vi "Check_Execution_Row.vi"(0 "Execution Row":T1 {"Row Duration (mins)" format="%#.1f"; "Row No" min=0; "Trace Gas Concentration (%)" min=0.0 format="%#.2f"; "Emission Rate (l/min)" format="%#.2f"; "Tunnel Speed" format="%#.2f"; "Start X" format="%#.2f"; "Start Y" format="%#.2f"; "Start Z" format="%#.2f"; "End X" format="%#.2f"; "End Y" format="%#.2f"; "End Z" format="%#.2f"; "Averaging time (min)" min=0.0 format="%#.2f"}, 3 "Synchronization Start No":i32=1 min=1 max=100, 4 "Row Index":i32, 5 "Max Tunnel Speed":dbl format="%.2f") -> (6 "Editted Row":bool, 7 "Execution Row Out":T1 {"Row Duration (mins)" format="%#.1f"; "Row No" min=0; "Trace Gas Concentration (%)" min=0.0 format="%#.2f"; "Emission Rate (l/min)" format="%#.2f"; "Tunnel Speed" format="%#.2f"; "Start X" format="%#.2f"; "Start Y" format="%#.2f"; "Start Z" format="%#.2f"; "End X" format="%#.2f"; "End Y" format="%#.2f"; "End Z" format="%#.2f"; "Averaging time (min)" min=0.0 format="%#.2f"}, 9 "Continue?":bool, 10 "Error Comments":string)   [LabVIEW 2010]
uses:
  Traverse_cluster.ctl
  Spacing.ctl
  Controls/Multi_run_mode.ctl
  Controls/User_Specific_mode.ctl
  Controls/Tunnel_Coordinates.ctl
  ADAM Client/Sub VIs/ADAM Controls/Channel_names.ctl
  Globals/Extra_Commands_Global.vi
  Globals/Constants_global.vi
  Globals/Trav_pos_global.vi
panel:
  out "Fixed Axis":bool[](array[boolean])
  out "Filenames":string[](array[string])
  out "Current Sync Number":i32
  out "Checks":string[](array[string])
  in  "Edit in Excel":bool
  in  "OK":bool
  # "X           Y            Z"
  # "Start"
  # "End"
  # "X           Y            Z"
  # "Start"
  # "End"
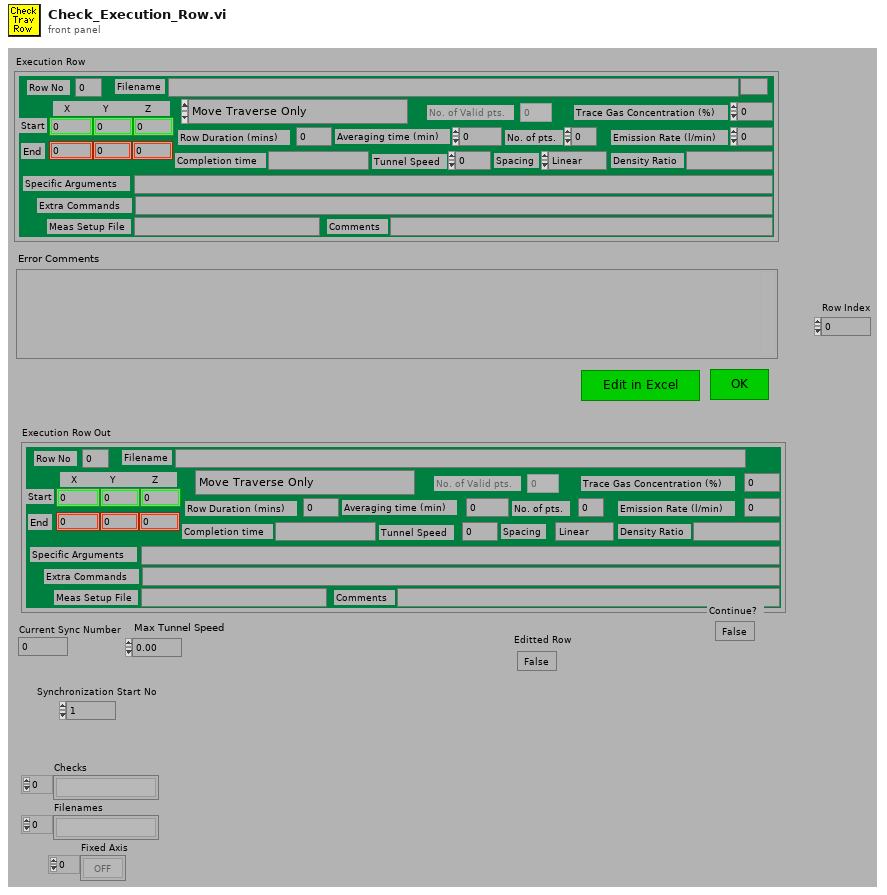
[diagram p1: front panel]
types:
  T1 = typedef "Traverse_cluster.ctl" = cluster{"Start X":dbl, "Start Y":dbl, "Start Z":dbl, "End X":dbl, "End Y":dbl, "End Z":dbl, "No. of pts.":i32, "Spacing":T2, "Filename":path, "Tunnel Speed":dbl, "Averaging time (min)":dbl, "Extra Commands":string, "Specific Arguments":string, "Emission Rate (l/min)":dbl, "Trace Gas Concentration (%)":dbl, "Density Ratio":string, "Comments":string, "Row No":i32, "Row Type Selector":T3, "Completion time":string, "Row Duration (mins)":dbl, "No. of Valid pts.":i32, "Meas Setup File":string}
  T2 = typedef "Spacing.ctl" = enum16{"Linear", "Log", "Gauss", "Specified", "N/A"}
  T3 = typedef "Multi_run_mode.ctl" = enum16{"Move Traverse Only", "Set Tunnel Speed Only", "Set Source Only", "Set Measurement Conditions", "Single Measurement", "Vertical Profile", "Lateral Profile", "Longitudinal Profile", "Explore Volume", "Multi-Axis Profile", "Auto Calibrate", "Meas Fast FID Bkgnd", "Check Beam Power", "Scanning Valve Measurement", "Run VI Named:", "Set ADAM Ch", "Wait (minutes)", "Send Message", "Synchronize With:", "Fall Back to this Row", "Turn Off Row Repeating", "Blank Row"}
  T4 = enum16{"All Channel Names", "Valid Channel Names"}
  T5 = typedef "User_Specific_mode.ctl" = enum16{"Check VI only", "Run VI"}
  T6 = typedef "Tunnel_Coordinates.ctl" = enum16{"Work in Tunnel Coordinates", "Work in Model Coordinates"}
  T7 = enum16{"Zero or one", "One", "Zero or more", "One or more"}
  T8 = typedef "Channel_names.ctl" = enum16{"Active Only", "Active + Off", "All Channels"}
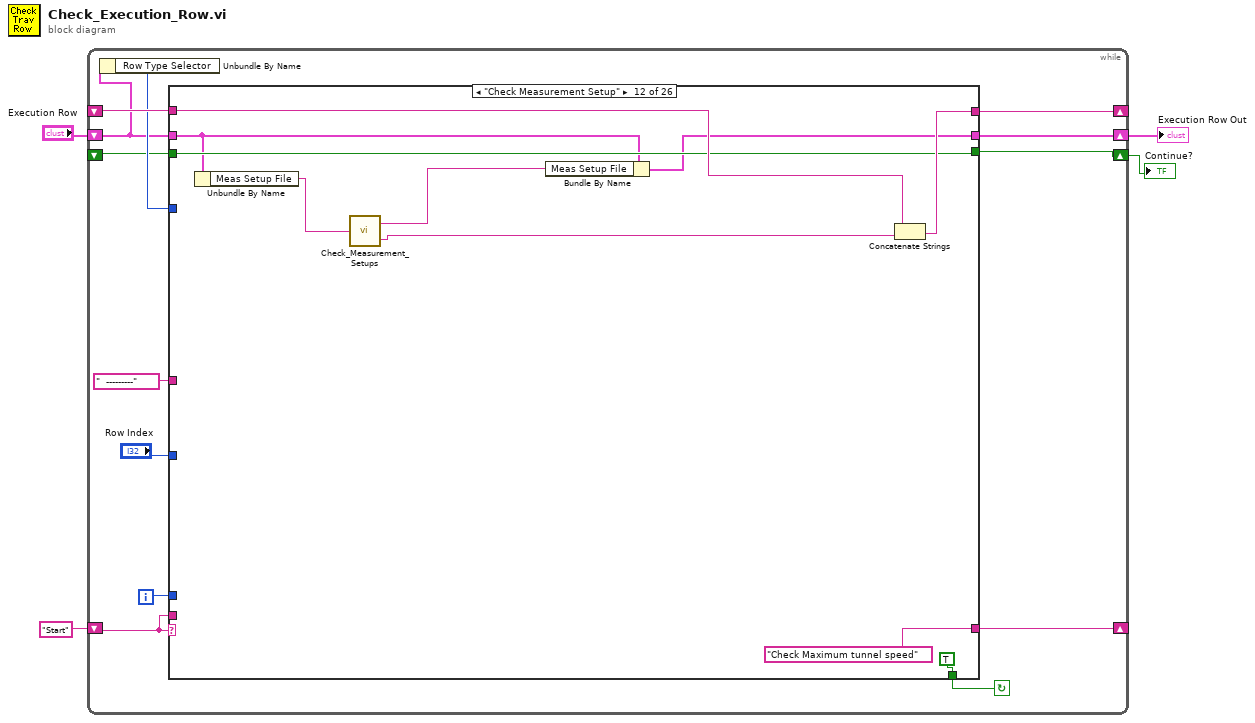
[diagram p0: block diagram]
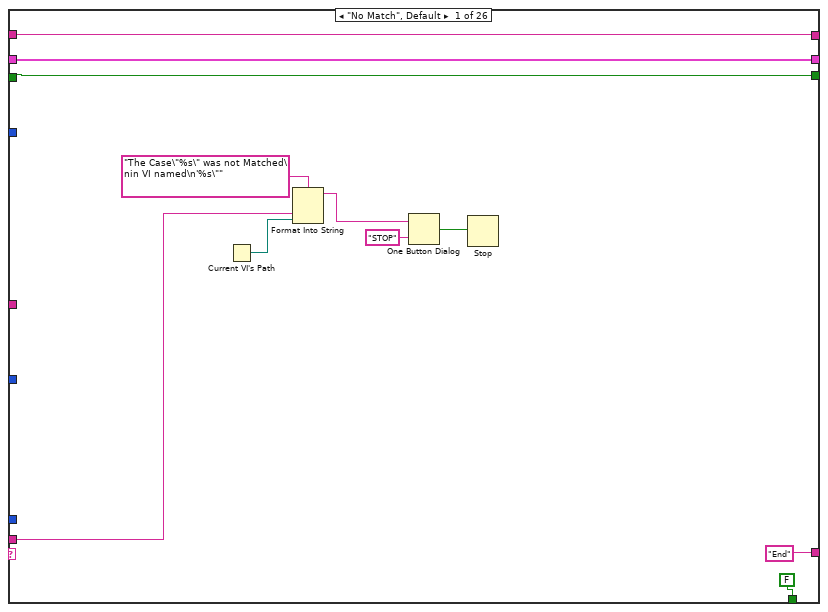
[diagram p2: hidden frame]
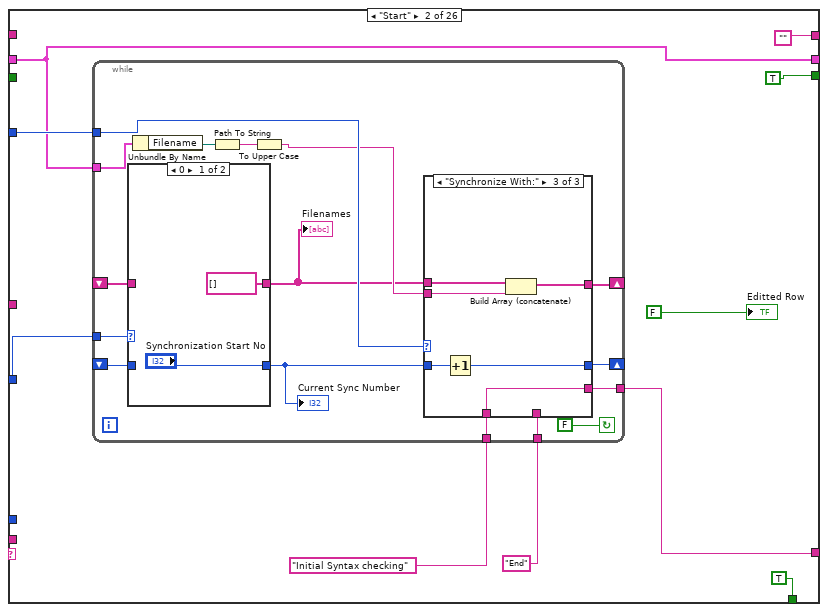
[diagram p3: hidden frame]
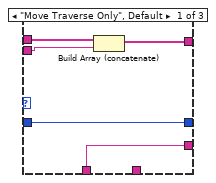
[diagram p5: hidden frame]
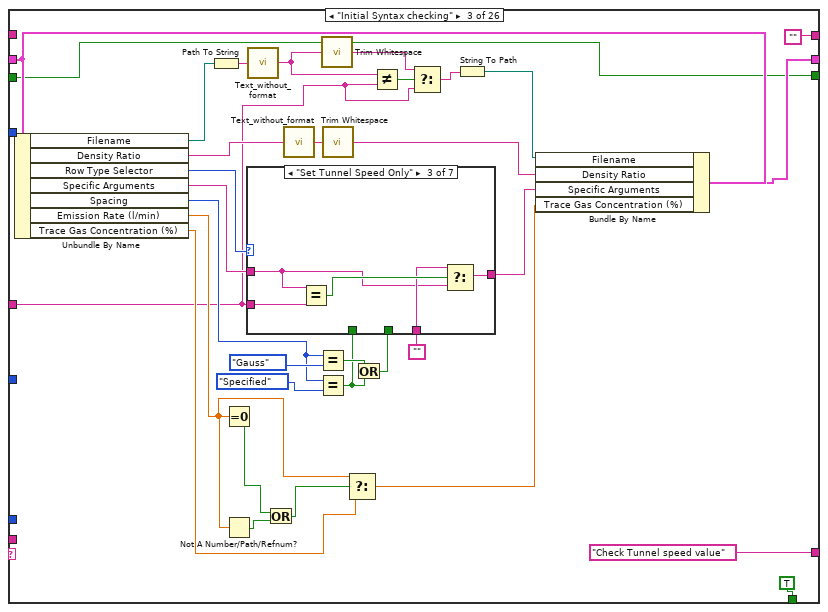
[diagram p7: hidden frame]
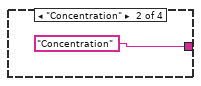
[diagram p10: hidden frame]
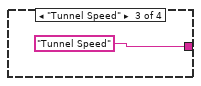
[diagram p11: hidden frame]
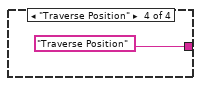
[diagram p12: hidden frame]
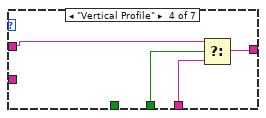
[diagram p13: hidden frame]
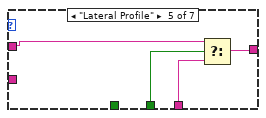
[diagram p14: hidden frame]
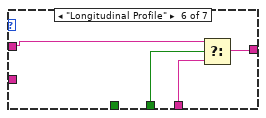
[diagram p15: hidden frame]
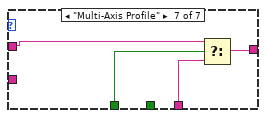
[diagram p16: hidden frame]
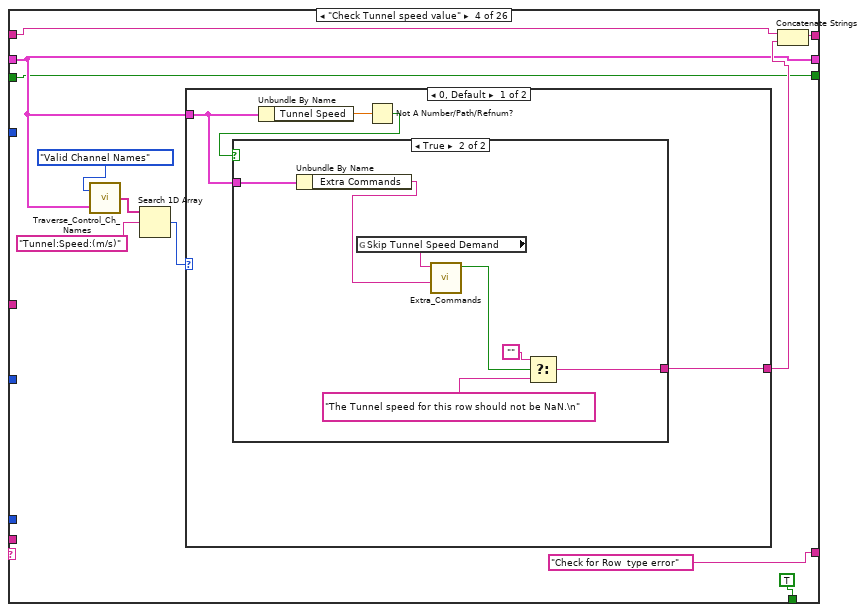
[diagram p17: hidden frame]
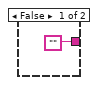
[diagram p18: hidden frame]
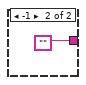
[diagram p19: hidden frame]
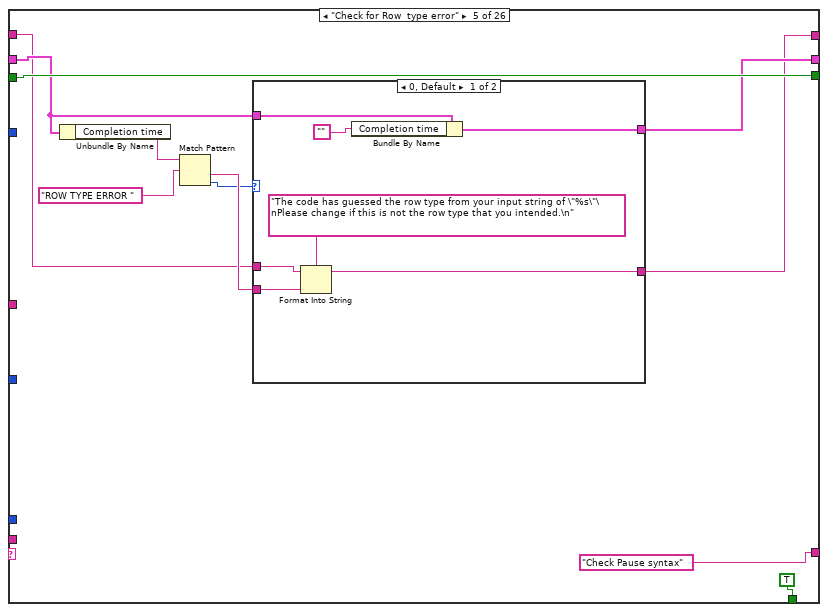
[diagram p20: hidden frame]
diagram:
  n1 = while {
    shift-left: _ -> [w16]
    shift-right: [w17] -> _
    shift-left: "Start" -> [w9]
    shift-right: [w14] -> _
    shift-right: [w8] -> w2
    shift-left: "Execution Row" -> [w5]
    shift-right: [w7] -> w1
    shift-left: _ -> [w6]
    i -> [w10]
    stop <- w15 continue-if-true
    n2 = Unbundle By Name(w5) -> ("Row Type Selector"=w12:T3)
    n3 = case shown="\"Check Measurement Setup\"" w9 {
      tunnel: w5 -> [w22 w32 w100 w137 w161 w191 w204 w252 w283 w313 w369 w401 w409 w448 w779 w879 w916 w938 w1022 w1054 w1064 w1133 _ w1172 w1179 w1189]
      tunnel: "  ---------" ("f") -> [_ _ w74 _ _ w195 _ _ _ _ _ _ _ _ _ _ _ _ _ _ _ _ _ _ _ _]
      tunnel: "Row Index" -> [_ w36 _ _ _ _ w201 _ _ _ _ _ _ w442 _ _ _ _ _ _ _ _ _ w1173 _ w1188]
      tunnel: [w21 "" "" w138 w158 w183 w218 w254 w288 w318 w371 w405 w414 w452 w784 w889 w922 w963 w1020 w1058 w1065 w1139 w1150 w1174 w1184 w1191] -> w17
      tunnel: w12 -> [_ w35 _ _ _ _ w209 _ _ _ _ _ w412 w451 w780 w877 _ _ _ _ w1069 _ _ _ _ _]
      tunnel: w16 -> [w21 _ _ w139 w159 w185 w219 w255 w289 w319 w371 w404 w415 w453 w784 w890 w923 w964 w1020 w1059 w1070 w1139 w1150 w1174 w1184 w1191]
      tunnel: [FALSE TRUE TRUE TRUE TRUE TRUE TRUE TRUE TRUE TRUE TRUE TRUE TRUE TRUE TRUE TRUE TRUE TRUE TRUE TRUE w1061 TRUE TRUE TRUE TRUE FALSE] -> w15
      tunnel: ["End" w33 "Check Tunnel speed value" ("f") "Check for Row  type error" ("f") "Check Pause syntax" ("f") w188 w206 "Check Traverse Setup Name" ("f") "Check IF command" ("f") "Check Measurement Setup?" ("f") w373 "Check Maximum tunnel speed" ("f") "Row type specific check" ("f") w449 "Check for position NaNs" ("f") w880 "Check source details" ("t") "Check source details" ("f") w1017 "check entered filename etc" ("f") w1067 "What to do next?" ("f") w1148 "Initial Syntax checking" "End" "End"] -> w14
      tunnel: w10 -> [_ _ _ _ _ _ _ _ _ _ _ _ _ _ _ _ _ _ _ _ _ _ _ _ _ _]
      tunnel: w9 -> [w23 _ _ _ _ _ _ _ _ _ _ _ _ _ _ _ _ _ _ _ _ _ _ _ _ _]
      tunnel: [w22 w32 w77 w137 w162 w178 w203 w252 w283 w313 w369 w400 w409 w443 w778 w879 w916 w937 w1021 w1054 w1063 w1133 w1141 w1175 w1179 w1187] -> w8
      tunnel: [w18 TRUE w75 w136 w168 w179 w205 w248 w280 w310 w375 w402 w407 w445 w776 w878 w915 w935 w1025 w1052 w1061 w1132 w1140 w1169 w1178 w1185] -> w7
      tunnel: w6 -> [w18 _ w75 w136 w168 w179 w205 w248 w280 w310 w375 w402 w407 w445 w776 w878 w915 w935 w1025 w1052 _ w1132 _ w1169 w1178 w1185]
      frame "No Match", Default {
        n4 = Current VI's Path() -> (path=w24:path)
        n5 = Format Into String(format string="The Case\"%s\" was not Matched\nin VI named\n'%s\"" ("Format String"), w23, w24) -> (resulting string=w27:string)  [unwired: 2 in, 1 out]
        n6 = One Button Dialog(message=w27, button name ("OK")="STOP") -> (true=w25:bool)
        n7 = Stop(stop? (T)=w25) -> ()
      }
      frame "Start" {
        n8 = while {
          tunnel: "End" -> [w40]
          tunnel: "Initial Syntax checking" -> [w41]
          tunnel: [w42] -> w33
          tunnel: w32 -> [w49]
          shift-left: _ -> [w48]
          shift-right: [w47] -> _
          tunnel: w35 -> [w53]
          shift-left: _ -> [w52]
          shift-right: [w51] -> _
          tunnel: w36 -> [w54]
          stop <- FALSE continue-if-true
          n9 = case shown="0" w54 {
            tunnel: ["Synchronization Start No" w58] -> w50
            tunnel: w52 -> [_ w58]
            tunnel: w48 -> [_ w57]
            tunnel: [string[] [] w57] -> w43
            frame 0 {
            }
            frame 1, Default {
            }
          }
          "Current Sync Number" <- w50
          "Filenames" <- w43
          n10 = Unbundle By Name(w49) -> ("Filename"=w46:path)
          n11 = Path To String(path=w46) -> (string=w45:string)
          n12 = To Upper Case(1:w45) -> (0:w44:string)
          n13 = case shown="\"Synchronize With:\"" w53 {
            tunnel: w50 -> [w63 w66 w72]
            tunnel: [w63 w66 w71] -> w51
            tunnel: w44 -> [w61 _ w70]
            tunnel: w43 -> [w62 w65 w69]
            tunnel: [w60 w65 w68] -> w47
            tunnel: [w59 w64 w67] -> w42
            tunnel: w41 -> [w59 _ w67]
            tunnel: w40 -> [_ w64 _]
            frame "Move Traverse Only", Default {
              n14 = Build Array (concatenate)(w62, w61) -> (w60:string[])
            }
            frame "Blank Row" {
            }
            frame "Synchronize With:" {
              n15 = Increment(x=w72) -> (x+1=w71:i32)
              n16 = Build Array (concatenate)(w69, w70) -> (w68:string[])
            }
          }
        }
        "Editted Row" <- FALSE ("Editted Row")
      }
      frame "Initial Syntax checking" {
        n17 = Unbundle By Name(w100) -> ("Filename"=w73:path, "Density Ratio"=w79:string, "Row Type Selector"=w97:T3, "Specific Arguments"=w95:string, "Spacing"=w87:T2, "Emission Rate (l/min)"=w83:dbl, "Trace Gas Concentration (%)"=w93:dbl)
        n18 = Path To String(path=w73) -> (string=w81:string)
        n19 = Equal To 0?(x=w83) -> (x = 0?=w85:bool)
        n20 = Not A Number/Path/Refnum?(number/path/refnum=w83) -> (NaN/Path/Refnum?=w84:bool)
        n21 = call "Text_without_format.vi"("Input string"=w81) -> ("Output string"=w104:string)
        n22 = Or(x=w85, y=w84) -> (x .or. y?=w82:bool)
        n23 = call "Text_without_format.vi"("Input string"=w79) -> ("Output string"=w99:string)
        n24 = Equal?(x=w87, y=Spacing."Gauss" ("Spacing")) -> (x = y?=w89:bool)
        n25 = Equal?(x=w87, y=Spacing."Specified" ("Spacing")) -> (x = y?=w86:bool)
        n26 = call <vilib>:"Trim Whitespace.vi"("string"=w104) -> ("trimmed string"=w103:string)  [unwired: 1 in]
        n27 = call <vilib>:"Trim Whitespace.vi"("string"=w99) -> ("trimmed string"=w78:string)  [unwired: 1 in]
        n28 = Select(t=w83, s=w82, f=w93) -> (s? t:f=w92:dbl)
        n29 = Or(x=w89, y=w86) -> (x .or. y?=w88:bool)
        n30 = case shown="\"Set Tunnel Speed Only\"" w97 {
          tunnel: [w106 w108 w113 w119 w123 w127 w131] -> w96
          tunnel: w95 -> [w106 w107 w114 w121 w125 w129 w133]
          tunnel: "" -> [_ _ w115 w120 w124 w128 w132]
          tunnel: w88 -> [_ _ _ w118 w122 w126 _]
          tunnel: w86 -> [_ _ _ _ _ _ w130]
          tunnel: w74 -> [_ _ w117 _ _ _ _]
          frame "Move Traverse Only", Default {
          }
          frame "Auto Calibrate" {
            n31 = case shown="\"No Match\", Default" w107 {
              tunnel: [w109 "Concentration" "Tunnel Speed" "Traverse Position"] -> w108
              tunnel: w107 -> [w109 _ _ _]
              frame "No Match", Default {
              }
              frame "Concentration" {
              }
              frame "Tunnel Speed" {
              }
              frame "Traverse Position" {
              }
            }
          }
          frame "Set Tunnel Speed Only" {
            n32 = Equal?(x=w114, y=w117) -> (x = y?=w116:bool)
            n33 = Select(t=w115, s=w116, f=w114) -> (s? t:f=w113:string)
          }
          frame "Vertical Profile" {
            n34 = Select(t=w121, s=w118, f=w120) -> (s? t:f=w119:string)
          }
          frame "Lateral Profile" {
            n35 = Select(t=w125, s=w122, f=w124) -> (s? t:f=w123:string)
          }
          frame "Longitudinal Profile" {
            n36 = Select(t=w129, s=w126, f=w128) -> (s? t:f=w127:string)
          }
          frame "Multi-Axis Profile" {
            n37 = Select(t=w133, s=w130, f=w132) -> (s? t:f=w131:string)
          }
        }
        n38 = Not Equal?(x=w104, y=w74) -> (x != y?=w105:bool)
        n39 = Select(t=w103, s=w105, f=w74) -> (s? t:f=w102:string)
        n40 = String To Path(string=w102) -> (path=w80:path)
        n41 = Bundle By Name(cluster=w100, "Filename"=w80, "Density Ratio"=w78, "Specific Arguments"=w96, "Trace Gas Concentration (%)"=w92) -> (w77:T1)
      }
      frame "Check Tunnel speed value" {
        n42 = call "Traverse_Control_Ch_Names.vi"("Traverse line"=w137, "Mode"=T4."Valid Channel Names") -> ("Channel names"=w143:string[])
        n43 = Search 1D Array(1D array=w143, element="Tunnel:Speed:(m/s)" ("Label for value")) -> (index of element=w141:i32)  [unwired: 1 out]
        n44 = case shown="0, Default" w141 {
          tunnel: w137 -> [w146 _]
          tunnel: [w145 ""] -> w140
          frame 0, Default {
            n45 = Unbundle By Name(w146) -> ("Tunnel Speed"=w148:dbl)
            n46 = Not A Number/Path/Refnum?(number/path/refnum=w148) -> (NaN/Path/Refnum?=w147:bool)
            n47 = case shown="True" w147 {
              tunnel: w146 -> [_ w156]
              tunnel: ["" w150] -> w145
              frame False {
              }
              frame True {
                n48 = Unbundle By Name(w156) -> ("Extra Commands"=w154:string)
                n49 = global read "Extra_Commands_Global.vi" "Skip Tunnel Speed Demand"() -> (w155:string)
                n50 = call "Extra_Commands.vi"("String to Search"=w154, "Command"=w155) -> ("Command Found"=w153:bool)  [unwired: 1 in, 4 out]
                n51 = Select(t="", s=w153, f="The Tunnel speed for this row should not be NaN.\n") -> (s? t:f=w150:string)
              }
            }
          }
          frame -1 {
          }
        }
        n52 = Concatenate Strings(w139, w140) -> (w138:string)
      }
      frame "Check for Row  type error" {
        n53 = Unbundle By Name(w161) -> ("Completion time"=w164:string)
        n54 = Match Pattern(string=w164, regular expression="ROW TYPE ERROR " ("format string")) -> (after substring=w163:string, offset past match=w160:i32)  [unwired: 3 out]
        n55 = case shown="0, Default" w160 {
          tunnel: w163 -> [w175 _]
          tunnel: [w173 w177] -> w162
          tunnel: w161 -> [w172 w177]
          tunnel: [w170 w176] -> w158
          tunnel: w159 -> [w169 w176]
          frame 0, Default {
            n56 = Format Into String(format string="The code has guessed the row type from your input string of \"%s\"\nPlease change if this is not the row type that you intended.\n", initial string=w169, w175) -> (resulting string=w170:string)  [unwired: 1 in, 1 out]
            n57 = Bundle By Name(cluster=w172, "Completion time"="") -> (w173:T1)
          }
          frame -1 {
          }
        }
      }
      frame "Check Pause syntax" {
        n58 = Unbundle By Name(w191) -> ("Extra Commands"=w196:string)
        n59 = Not Equal?(x=w196, y=w195) -> (x != y?=w197:bool)
        n60 = Select(t=w196, s=w197, f="") -> (s? t:f=w193:string)
        n61 = call <vilib>:"Trim Whitespace.vi"("string"=w193) -> ("trimmed string"=w187:string)  [unwired: 1 in]
        n62 = Equal?(x=w187, y="") -> (x = y?=w189:bool)
        n63 = call "Pause_for_server_ch_val.vi"("Extra command string"=w187, "Simulate/Run"=User_Specific_mode."Check VI only") -> ("Extra command string Out"=w186:string, "Error Comments"=w184:string)
        n64 = Bundle By Name(cluster=w191, "Extra Commands"=w186) -> (w178:T1)
        n65 = Concatenate Strings(w185, w184) -> (w183:string)
        n66 = Select(t="Check Measurement Setup?", s=w189, f="Check Extra Commands") -> (s? t:f=w188:string)
      }
      frame "Check Extra Commands" {
        n67 = Unbundle By Name(w204) -> ("Extra Commands"=w212:string)
        n68 = for {
          N: 4 -> [_]
          tunnel: w212 -> [w227]
          shift-right: [w223] -> w215
          shift-left: "" -> [w224]
          i -> [w229]
          n69 = case shown="0, Default" w229 {
            tunnel: [w232 w234 w236 w238] -> w226
            tunnel: ["The Extra Command \"%s\" should have a numeric argument.\n" ("Format String") "The Extra Command \"%s\" should have a numeric argument.\n" ("Format String") "The Extra Command \"%s\" should have a numeric argument.\n" ("Format String") "The Extra Command \"%s\" should have a numeric argument.\n" ("Format String")] -> w221
            frame 0, Default {
              n70 = global read "Extra_Commands_Global.vi" "Coil Analysis time (s)"() -> (w232:string)
            }
            frame 1 {
              n71 = global read "Extra_Commands_Global.vi" "Estimated Av Csample/Csource"() -> (w234:string)
            }
            frame 2 {
              n72 = global read "Extra_Commands_Global.vi" "Establish Exp Conditions (s)"() -> (w236:string)
            }
            frame 3 {
              n73 = global read "Extra_Commands_Global.vi" "Minutes Before Repeating Row"() -> (w238:string)
            }
          }
          n74 = call "Extra_Commands.vi"("String to Search"=w227, "Command"=w226) -> ("String Value"=w228:string, "Command Found"=w230:bool)  [unwired: 1 in, 3 out]
          n75 = case shown="False" w230 {
            tunnel: w228 -> [_ w247]
            tunnel: w226 -> [_ w245]
            tunnel: [w239 w242] -> w225
            tunnel: "" -> [w239 w241]
            tunnel: w221 -> [_ w240]
            frame False {
            }
            frame True {
              n76 = Decimal String To Number(string=w247) -> (offset past number=w246:i32)  [unwired: 3 out]
              n77 = Equal To 0?(x=w246) -> (x = 0?=w244:bool)
              n78 = Format Into String(format string=w240, w245) -> (resulting string=w243:string)  [unwired: 2 in, 1 out]
              n79 = Select(t=w243, s=w244, f=w241) -> (s? t:f=w242:string)
            }
          }
          n80 = Concatenate Strings(w225, w224) -> (w223:string)
        }
        n81 = call "Trav_Prog_Extra_Commands.vi"() -> ("Extra Commands Array"=w213:string[])  [unwired: 2 out]
        n82 = call "Valid_Extra_Command.vi"("Extra Commands string"=w212, "Valid Commands Array"=w213) -> ("Output String"=w217:string, "Extra Commands string Out"=w202:string)  [unwired: 3 out]
        n83 = Bundle By Name(cluster=w204, "Extra Commands"=w202) -> (w203:T1)
        n84 = Equal?(x=w209, y=Multi_run_mode."Run VI Named:" ("Row Type Selector")) -> (x = y?=w208:bool)
        n85 = call "Skip_If Sd_Error_Below.vi"("String to Search"=w202, "Simulate/Run"=User_Specific_mode."Check VI only", "Measurement setup Applied?"=FALSE, "Row Number"=w201) -> ("Error String"=w198:string)  [unwired: 1 in, 4 out]
        n86 = Select(t="Check Release Script" ("f"), s=w208, f="Check Traverse Setup Name") -> (s? t:f=w206:string)
        n87 = Concatenate Strings(w219, w217, w215, w198) -> (w218:string)
      }
      frame "Check Release Script" {
        n88 = call "Get_Script_filename.vi"("Traverse line"=w252) -> ("Script Filename"=w250:path)
        n89 = call "Does_file_exist_(simple).vi"("Pathname"=w250) -> ("exists?"=w251:bool)
        n90 = case shown="False" w251 {
          tunnel: [w262 ""] -> w249
          tunnel: w250 -> [w260 _]
          frame False {
            n91 = Strip Path(path=w260) -> (stripped path=w261:path)  [unwired: 1 out]
            n92 = call "List_files_in_order_of_age.vi"("Folder"=w261) -> ("file names"=w266:string[])  [unwired: 1 in]
            n93 = Array Subset(array=w266, length=25 ("Array Length")) -> (w259:string[])  [unwired: 1 in]
            n94 = for {
              shift-right: [w269] -> w263
              shift-left: "" -> [w270]
              tunnel: w259 -> [w268] mode=indexing
              n95 = case shown="\"Calib Setup\"" w268 {
                tunnel: w268 -> [w274 _ _]
                tunnel: w270 -> [w271 w275 w276]
                tunnel: [w273 w275 w276] -> w269
                frame "False", Default {
                  n96 = Concatenate Strings(w271, w274, "      " ("Substring")) -> (w273:string)
                }
                frame "Current Setup" {
                }
                frame "Calib Setup" {
                }
              }
            }
            n97 = Index Array(array=w259, index=0) -> (element=w257:string)
            n98 = Format Into String(format string="The Gas Desk Release Script file \"%s\" does not exist.\n Valid filenames are: \n%s\nExample:  !Release Script Filename = %s\n" ("Format String"), w260, w263, w257) -> (resulting string=w262:string)  [unwired: 2 in, 1 out]
          }
          frame True {
          }
        }
        n99 = Concatenate Strings(w255, w249) -> (w254:string)
      }
      frame "Check Traverse Setup Name" {
        n100 = Unbundle By Name(w283) -> ("Extra Commands"=w279:string)
        n101 = global read "Extra_Commands_Global.vi" "!Traverse Setup"() -> (w286:string)
        n102 = call "Extra_Commands.vi"("String to Search"=w279, "Command"=w286) -> ("String Value"=w284:string, "Command Found"=w285:bool)  [unwired: 1 in, 3 out]
        n103 = case shown="True" w285 {
          tunnel: w284 -> [_ w296]
          tunnel: [w290 w293] -> w281
          tunnel: "" -> [w290 w292]
          frame False {
          }
          frame True {
            n104 = global read "Constants_global.vi" "Traverse folder"() -> (w291:path)
            n105 = List Folder(path=w291) -> (folder names=w294:string[])  [unwired: 1 in, 5 out]
            n106 = Search 1D Array(1D array=w294, element=w296) -> (index of element=w297:i32)  [unwired: 1 out]
            n107 = Greater Or Equal To 0?(x=w297) -> (x >= 0?=w295:bool)
            n108 = case shown="False" w295 {
              tunnel: w296 -> [w302 _]
              tunnel: w294 -> [w299 _]
              tunnel: [w298 w307] -> w293
              tunnel: w292 -> [_ w307]
              frame False {
                n109 = Format Into String(format string="%s is not a valid Travese setup. Valid option are:", w302) -> (resulting string=w300:string)  [unwired: 2 in, 1 out]
                n110 = for {
                  shift-right: [w304] -> w298
                  shift-left: w300 -> [w305]
                  tunnel: w299 -> [w306] mode=indexing
                  w303 = "  " ("Substring")
                  n111 = Concatenate Strings(w305, w303, w306, w303) -> (w304:string)
                }
              }
              frame True {
              }
            }
          }
        }
        n112 = Concatenate Strings(w289, w281) -> (w288:string)
      }
      frame "Check IF command" {
        n113 = Unbundle By Name(w313) -> ("Extra Commands"=w309:string)
        n114 = global read "Extra_Commands_Global.vi" "If Command"() -> (w316:string)
        n115 = call "Extra_Commands.vi"("String to Search"=w309, "Command"=w316) -> ("String Value"=w314:string, "Command Found"=w315:bool)  [unwired: 1 in, 3 out]
        n116 = case shown="True" w315 {
          tunnel: w314 -> [_ w325]
          tunnel: [w320 w324] -> w311
          tunnel: "" -> [w320 w322]
          frame False {
          }
          frame True {
            n117 = call "Get_array_values_fr_String.vi"("String Value"=w325) -> ("Numeric Array"=w321:dbl[], "String array"=w323:string[])
            n118 = Index Array(array=w323, index=0 ("Index")) -> (element=w326:string)
            n119 = case shown="\"Global Value Between\"" w326 {
              tunnel: w325 -> [w331 _ _ _]
              tunnel: [w330 w356 w357 "The !If  command has not been recognised.\nExtra command Example:\n!IF = Time Between;10:45;and;14:00;Execute Row (or) Skip Row\n\n!IF = ADAM Channel Between;Channel Name; 0.5;1.0\n\n!IF = Global Value Between; 0.5;1.0" ("Error Comments")] -> w324
              tunnel: w323 -> [_ w347 w365 _]
              tunnel: w322 -> [_ w340 w358 _]
              tunnel: w321 -> [_ _ _ _]
              frame "Time Between" {
                n120 = Get Date/Time In Seconds() -> (seconds since 1Jan1904=w328:timestamp)
                n121 = To Double Precision Float(number=w328) -> (double precision float=w329:dbl)
                n122 = call "If_Time_arguments.vi"("seconds since 1Jan1904"=w329, "String Value"=w331) -> ("Error Comments"=w330:string)  [unwired: 2 out]
              }
              frame "ADAM Channel Between" {
                n123 = Index Array(array=w347, index=1 ("Index")) -> (element=w350:string)
                n124 = Index Array(array=w347, index=2 ("Index")) -> (element=w346:string)
                n125 = Index Array(array=w347, index=3 ("Index")) -> (element=w345:string)
                n126 = Build Array(w350) -> (w352:string[])
                n127 = Decimal Digit?(1:w346) -> (0:w343:bool)
                n128 = Decimal Digit?(1:w345) -> (0:w344:bool)
                n129 = call "Get_Current_Scan_client.vi"("ADAM Ch Names"=w352) -> ("Numerical Values"=w354:dbl[])  [unwired: 3 out]
                n130 = And(x=w343, y=w344) -> (x .and. y?=w342:bool)
                n131 = Index Array(array=w354, index=0 ("Index")) -> (element=w355:dbl)
                n132 = Select(t=w340, s=w342, f="you must give two limits\n") -> (s? t:f=w336:string)
                n133 = Not A Number/Path/Refnum?(number/path/refnum=w355) -> (NaN/Path/Refnum?=w339:bool)
                n134 = Select(t="Invalid ADAM Channel Name\n", s=w339, f=w340) -> (s? t:f=w337:string)
                n135 = Concatenate Strings(w337, w336) -> (w334:string)
                n136 = Concatenate Strings(w334, "Extra command Example:\n!IF = ADAM Channel Between;Channel Name; 0.5;1.0") -> (w333:string)
                n137 = Empty String/Path?(string/path=w334) -> (empty?=w335:bool)
                n138 = Select(t=w340, s=w335, f=w333) -> (s? t:f=w356:string)
              }
              frame "Global Value Between" {
                n139 = Index Array(array=w365, index=1 ("Index")) -> (element=w364:string)
                n140 = Index Array(array=w365, index=2 ("Index")) -> (element=w363:string)
                n141 = Decimal Digit?(1:w364) -> (0:w361:bool)
                n142 = Decimal Digit?(1:w363) -> (0:w362:bool)
                n143 = And(x=w361, y=w362) -> (x .and. y?=w360:bool)
                n144 = Select(t=w358, s=w360, f="The Extra command IF statement must have two numerical values for the limits\n\nExtra command Example:\n!IF = Global Value Between; 0.5;1.0") -> (s? t:f=w357:string)
              }
              frame "No Match", Default {
              }
            }
          }
        }
        n145 = Concatenate Strings(w319, w311) -> (w318:string)
      }
      frame "Check Measurement Setup?" {
        n146 = Unbundle By Name(w369) -> ("Row Type Selector"=w374:T3, "Specific Arguments"=w372:string)
        n147 = case shown="\"Lateral Profile\"" w374 {
          tunnel: ["Check Measurement Setup" ("t") "Check Measurement Setup" ("t") "Check Measurement Setup" ("t") "Check Measurement Setup" ("t") "Check Measurement Setup" ("t") "Check Measurement Setup" ("t") "Check Measurement Setup" ("t") "Check Measurement Setup" ("t") "Check Measurement Setup" ("t") "Check Measurement Setup" ("t") w387 w396] -> w373
          tunnel: w372 -> [_ _ _ _ _ _ _ _ _ _ w394 _]
          tunnel: "Check Maximum tunnel speed" ("f") -> [_ _ _ _ _ _ _ _ _ _ w388 w396]
          tunnel: w369 -> [_ _ _ _ _ _ _ _ _ _ w391 _]
          frame "Lateral Profile" {
          }
          frame "Longitudinal Profile" {
          }
          frame "Explore Volume" {
          }
          frame "Multi-Axis Profile" {
          }
          frame "Vertical Profile" {
          }
          frame "Single Measurement" {
          }
          frame "Scanning Valve Measurement" {
          }
          frame "Auto Calibrate" {
          }
          frame "Meas Fast FID Bkgnd" {
          }
          frame "Check Beam Power" {
          }
          frame "Run VI Named:" {
            n148 = Match Pattern(string=w394, regular expression=";") -> (before substring=w393:string)  [unwired: 4 out]
            n149 = call <vilib>:"Trim Whitespace.vi"("string"=w393) -> ("trimmed string"=w392:string)  [unwired: 1 in]
            n150 = call "Run_VI_Named_specific.vi"("Run VI Named String"=w392, "Multi Run Row"=w391) -> ("Check Meas Setup?"=w390:bool)  [unwired: 9 out]
            n151 = Select(t="Check Measurement Setup", s=w390, f=w388) -> (s? t:f=w387:string)
          }
          frame "Set Tunnel Speed Only", Default {
          }
        }
      }
      frame "Check Measurement Setup" {
        n152 = Unbundle By Name(w401) -> ("Meas Setup File"=w399:string)
        n153 = call "Check_Measurement_Setups.vi"("Measurement Setup String"=w399) -> ("Measurement Setup String Out"=w398:string, "Error Comments"=w397:string)
        n154 = Bundle By Name(cluster=w401, "Meas Setup File"=w398) -> (w400:T1)
        n155 = Concatenate Strings(w404, w397) -> (w405:string)
      }
      frame "Check Maximum tunnel speed" {
        n156 = case shown="\"Set Tunnel Speed Only\", Default" w412 {
          tunnel: w409 -> [w434 _]
          tunnel: [w425 FALSE] -> w411
          tunnel: [w424 0.0] -> w410
          frame "Auto Calibrate" {
            n157 = Unbundle By Name(w434) -> ("Specific Arguments"=w433:string)
            n158 = call "Get_array_values_fr_String.vi"("String Value"=w433) -> ("Numeric Array"=w427:dbl[], "String array"=w432:string[])
            n159 = Index Array(array=w432, index=0 ("Index")) -> (element=w430:string)
            n160 = Equal?(x=w430, y="Tunnel Speed" ("Output Array")) -> (x = y?=w425:bool)
            n161 = Array Subset(array=w427, index=1 ("Array Index")) -> (w426:dbl[])  [unwired: 1 in]
            n162 = Array Max & Min(array=w426) -> (max value=w424:dbl)  [unwired: 3 out]
          }
          frame "Set Tunnel Speed Only", Default {
          }
        }
        n163 = case shown="False" w411 {
          tunnel: [w422 w423] -> w419
          tunnel: w409 -> [w421 _]
          tunnel: w410 -> [_ w423]
          frame False {
            n164 = Unbundle By Name(w421) -> ("Tunnel Speed"=w422:dbl)
          }
          frame True {
          }
        }
        n165 = Greater?(x=w419, y="Max Tunnel Speed") -> (0:w417:bool)
        n166 = Not A Number/Path/Refnum?(number/path/refnum=w419) -> (NaN/Path/Refnum?=w418:bool)
        n167 = Compound Arithmetic op=AND(invert w418, w417) -> (w416:bool)
        n168 = case shown="False" w416 {
          tunnel: w415 -> [w437 w439]
          tunnel: [w437 w438] -> w414
          tunnel: "Max Tunnel Speed" -> [_ w441]
          frame False {
          }
          frame True {
            n169 = Format Into String(format string="The maximum allowable tunnel speed is %.2f m/s.\n" ("Format String"), initial string=w439, w441) -> (resulting string=w438:string)  [unwired: 1 in, 1 out]
          }
        }
      }
      frame "Row type specific check" {
        n170 = case shown="\"Auto Calibrate\"" w451 {
          tunnel: w448 -> [w462 w471 w475 w479 w484 w489 w496 w503 w514 w522 w548 w602 w609 w630 w658 w707 w735 w740 w744 w756 w760 w766]
          tunnel: [string[] [] string[] [] string[] [] string[] [] w485 w492 w499 w506 w519 w527 w556 w604 string[] [] w647 string[] [] w702 string[] [] string[] [] string[] [] string[] [] string[] [] string[] []] -> w450
          tunnel: [w456 "" "" "" "" "" "" "" w515 w524 w570 w598 w608 w642 w650 w718 w737 "" w746 "" "" w768] -> w454
          tunnel: [w465 w472 w476 w480 w483 w490 w497 w504 w513 w523 w555 w592 w607 w641 w661 w703 "check entered filename etc" "check entered filename etc" "check entered filename etc" "check entered filename etc" "check entered filename etc" "check entered filename etc"] -> w449
          tunnel: "Check source details" -> [_ w472 w476 _ _ _ _ _ _ _ _ w592 w607 w641 w660 w704 _ _ _ _ _ _]
          tunnel: "Sort out start and end positions" -> [_ _ _ _ _ w490 w497 w504 _ w523 w553 _ _ _ _ _ _ _ _ _ _ _]
          tunnel: "Check for Start NaNs" -> [w465 _ _ w480 w483 _ _ _ w513 _ w554 _ _ _ _ _ _ _ _ _ _ _]
          tunnel: [w461 w471 w475 w479 w484 w489 w496 w503 w514 w522 w534 w602 w617 w630 w657 w707 w735 w740 w744 w756 w760 w764] -> w443
          tunnel: w442 -> [_ _ _ _ _ _ _ _ _ _ _ _ _ _ w663 _ _ _ _ _ _ _]
          frame "Move Traverse Only" {
            n171 = Unbundle By Name(w462) -> ("Specific Arguments"=w463:string)
            n172 = call <vilib>:"Trim Whitespace.vi"("string"=w463) -> ("trimmed string"=w457:string)  [unwired: 1 in]
            n173 = Equal?(x=w457, y="No Backlash") -> (x = y?=w460:bool)
            n174 = Empty String/Path?(string/path=w457) -> (empty?=w459:bool)
            n175 = Or(x=w459, y=w460) -> (x .or. y?=w458:bool)
            n176 = case shown="True" w458 {
              tunnel: w457 -> [w468 _]
              tunnel: [w467 ""] -> w456
              frame False {
                n177 = Format Into String(format string="\"%s\" is an Incorrect Specific Argument. It should either be left blank or say \"No Backlash\"\n", w468) -> (resulting string=w467:string)  [unwired: 2 in, 1 out]
              }
              frame True {
              }
            }
            n178 = Bundle By Name(cluster=w462, "Specific Arguments"=w457) -> (w461:T1)
          }
          frame "Set Tunnel Speed Only" {
          }
          frame "Set Source Only" {
          }
          frame "Set Measurement Conditions" {
          }
          frame "Single Measurement" {
            n179 = Build Array("Averaging:Time:(mins)" ("Label for value"), "Filename:HD:Users" ("Label for value")) -> (w485:string[])
          }
          frame "Vertical Profile" {
            n180 = Build Array("Number:Of:Points" ("Label for value"), "Averaging:Time:(mins)" ("Label for value"), "Filename:HD:Users" ("Label for value")) -> (w492:string[])
          }
          frame "Lateral Profile" {
            n181 = Build Array("Number:Of:Points" ("Label for value"), "Averaging:Time:(mins)" ("Label for value"), "Filename:HD:Users" ("Label for value")) -> (w499:string[])
          }
          frame "Longitudinal Profile" {
            n182 = Build Array("Number:Of:Points" ("Label for value"), "Averaging:Time:(mins)" ("Label for value"), "Filename:HD:Users" ("Label for value")) -> (w506:string[])
          }
          frame "Explore Volume" {
            n183 = Unbundle By Name(w514) -> ("Specific Arguments"=w512:string)
            n184 = Build Array("Averaging:Time:(mins)" ("Label for value"), "Filename:HD:Users" ("Label for value")) -> (w519:string[])
            n185 = Fract/Exp String To Number(string=w512) -> (number=w511:dbl)  [unwired: 4 out]
            n186 = Greater Than 0?(x=w511) -> (x > 0?=w510:bool)
            n187 = Format Into String(format string="\"%s\" is an Incorrect Specific Argument. Please enter the radius of the volume in mm.\n", w512) -> (resulting string=w516:string)  [unwired: 2 in, 1 out]
            n188 = Select(t="", s=w510, f=w516) -> (s? t:f=w515:string)
          }
          frame "Multi-Axis Profile" {
            n189 = Unbundle By Name(w522) -> ("Spacing"=w525:T2)
            n190 = case shown="\"N/A\"" w525 {
              tunnel: ["" "You are not allowed to specify gaussian spacing for a Multi-Axis profile.\n" "You are not allowed to specify Log spacing for a Multi-Axis profile.\n" "\"N/A\" is not a valid point spacing.\n"] -> w524
              frame "Linear", Default {
              }
              frame "Gauss" {
              }
              frame "Log" {
              }
              frame "N/A" {
              }
            }
            n191 = Build Array("Number:Of:Points" ("Label for value"), "Averaging:Time:(mins)" ("Label for value"), "Filename:HD:Users" ("Label for value")) -> (w527:string[])
          }
          frame "Auto Calibrate" {
            n192 = Unbundle By Name(w548) -> ("Filename"=w537:path, "Specific Arguments"=w569:string)
            n193 = call "Get_array_values_fr_String.vi"("String Value"=w569) -> ("Numeric Array"=w565:dbl[], "String array"=w552:string[])
            n194 = global read "Trav_pos_global.vi" "Work in Tunnel Coordinates?"() -> (w547:T6)
            n195 = Index Array(array=w552, index=0 ("Index")) -> (element=w551:string)
            n196 = Build Array("Tunnel Speed", "Traverse Position", "Concentration") -> (w550:string[])
            n197 = Build Array("Averaging:Time:(mins)" ("Label for value")) -> (w556:string[])
            n198 = Array Size(array=w565) -> (size(s)=w564:i32)
            n199 = call "Current_Filepath.vi"("Filename in"=w537, "Data Type"="Calibrations") -> ("Filename Out"=w535:path)  [unwired: 1 out]
            n200 = Equal?(x=w547, y=Tunnel_Coordinates."Work in Model Coordinates" ("Work in Tunnel Coordinates?")) -> (x = y?=w541:bool)
            n201 = Search 1D Array(1D array=w550, element=w551) -> (index of element=w542:i32)  [unwired: 1 out]
            n202 = Equal?(x=2, y=w542) -> (x = y?=w544:bool)
            n203 = case shown="1" w542 {
              tunnel: [w590 w591] -> w555
              tunnel: w554 -> [w590 _]
              tunnel: w553 -> [_ w591]
              frame 0, Default {
              }
              frame 1 {
              }
            }
            n204 = Less?(x=w564, y=3) -> (x < y?=w560:bool)
            n205 = Equal To 0?(x=w542) -> (x = 0?=w561:bool)
            n206 = And(x=w541, y=w544) -> (x .and. y?=w543:bool)
            n207 = Greater Or Equal To 0?(x=w542) -> (x >= 0?=w540:bool)
            n208 = Compound Arithmetic op=AND(w560, w561) -> (w559:bool)
            n209 = case shown="True" w543 {
              tunnel: w548 -> [w586 w588]
              tunnel: [w586 w587] -> w536
              frame False {
              }
              frame True {
                n210 = Bundle By Name(cluster=w588, "Comments"="WARNING POSITION IN TUNNEL COORDINATES!!") -> (w587:T1)
              }
            }
            n211 = Select(t="You need to enter the desired tunnel speeds in the \"Specfic Arguments\" Box   eg.  Tunnel Speed;1;2;3;4\n", s=w559, f="") -> (s? t:f=w557:string)
            n212 = call "Does_file_exist_(simple).vi"("Pathname"=w535) -> ("exists?"=w575:bool)
            n213 = case shown="False" w540 {
              tunnel: w550 -> [w577 _]
              tunnel: [w576 ""] -> w539
              frame False {
                n214 = for {
                  shift-right: [w582] -> w579
                  shift-left: "Incorrect Specific Argument. The options are: " -> [w583]
                  tunnel: w577 -> [w584] mode=indexing
                  w581 = "  " ("Substring")
                  n215 = Concatenate Strings(w583, w581, w584, w581) -> (w582:string)
                }
                n216 = Concatenate Strings(w579, "\r") -> (w576:string)
              }
              frame True {
              }
            }
            n217 = Select(t="", s=w575, f="The calibration file cannot be found.\n") -> (s? t:f=w571:string)
            n218 = Bundle By Name(cluster=w536, "Filename"=w535) -> (w534:T1)
            n219 = Concatenate Strings(w571, w557, w539) -> (w570:string)
          }
          frame "Meas Fast FID Bkgnd" {
            n220 = Unbundle By Name(w602) -> ("Specific Arguments"=w597:string)
            n221 = call "Get_array_values_fr_String.vi"("String Value"=w597) -> ("String array"=w596:string[])  [unwired: 1 out]
            n222 = Index Array(array=w596, index=0) -> (element=w594:string)
            n223 = Empty String/Path?(string/path=w594) -> (empty?=w600:bool)
            n224 = Build Array("Averaging:Time:(mins)" ("Label for value")) -> (w604:string[])
            n225 = Equal?(x=w594, y="Use Source Divertor Valve") -> (x = y?=w593:bool)
            n226 = Or(x=w600, y=w593) -> (x .or. y?=w599:bool)
            n227 = case shown="False" w599 {
              tunnel: ["Specific Argument should either be blank or\nUse Source Divertor Valve ; (wait time in seconds optional)" ""] -> w598
              frame False {
              }
              frame True {
              }
            }
          }
          frame "Check Beam Power" {
            n228 = Unbundle By Name(w609) -> ("Extra Commands"=w611:string, "Start X"=w616:dbl, "Start Y"=w614:dbl, "Start Z"=w615:dbl)
            n229 = global read "Extra_Commands_Global.vi" "Skip Traverse Position Demand"() -> (w612:string)
            n230 = call "Extra_Commands.vi"("String to Search"=w611, "Command"=w612) -> ("Command Found"=w610:bool)  [unwired: 1 in, 4 out]
            n231 = case shown="False" w610 {
              tunnel: w616 -> [w628 _]
              tunnel: w615 -> [w627 _]
              tunnel: w614 -> [w626 _]
              tunnel: "" -> [w623 w629]
              tunnel: [w622 w629] -> w608
              frame False {
                n232 = Build Array(w628, w626, w627) -> (w625:dbl[])
                n233 = Not A Number/Path/Refnum?(number/path/refnum=w625) -> (NaN/Path/Refnum?=w624:bool[])
                n234 = Or Array Elements(Boolean array=w624) -> (logical OR=w621:bool)
                n235 = Select(t="The start position is where the datum velocity measurement will be made. This should not contain NaNs.\n" ("f"), s=w621, f=w623) -> (s? t:f=w622:string)
              }
              frame True {
              }
            }
            n236 = Bundle By Name(cluster=w609, "Comments"="Start Position is the location of Datum Velocity Measurement") -> (w617:T1)
          }
          frame "Scanning Valve Measurement" {
            w643 = ext -0.5  # lo
            w644 = ext 47.5  # hi
            n237 = Unbundle By Name(w630) -> ("Specific Arguments"=w640:string)
            n238 = call "Get_array_values_fr_String.vi"("String Value"=w640) -> ("Numeric Array"=w639:dbl[], "String array"=w635:string[])
            n239 = Build Array("Averaging:Time:(mins)" ("Label for value"), "Filename:HD:Users" ("Label for value")) -> (w647:string[])
            n240 = Index Array(array=w635, index=0) -> (element=w634:string)
            n241 = Empty String/Path?(string/path=w634) -> (empty?=w632:bool)
            n242 = Index Array(array=w639, index=0) -> (element=w637:dbl)
            n243 = In Range and Coerce(upper limit=w644, x=w637, lower limit=w643) -> (In Range?=w633:bool)  [unwired: 1 out]
            n244 = Compound Arithmetic op=AND(invert w632, w633) -> (w631:bool)
            n245 = Select(t="", s=w631, f="Enter the scanning valve port number between 0 and 47 in the specific arguments box.\n") -> (s? t:f=w642:string)
          }
          frame "Set ADAM Ch" {
            n246 = Unbundle By Name(w658) -> ("Specific Arguments"=w669:string)
            n247 = while {
              shift-right: [w697] -> w665
              shift-left: _ -> [w690]
              shift-right: [w696] -> _
              shift-left: _ -> [w695]
              tunnel: w663 -> [w696]
              stop <- TRUE stop-if-true
              n248 = Array Size(array=w690) -> (size(s)=w694:i32)
              n249 = Less?(x=w696, y=w695) -> (x < y?=w692:bool)
              n250 = Equal To 0?(x=w694) -> (x = 0?=w693:bool)
              n251 = Or(x=w693, y=w692) -> (x .or. y?=w691:bool)
              n252 = case shown="True" w691 {
                tunnel: [w698 w699] -> w697
                tunnel: w690 -> [w698 _]
                frame False {
                }
                frame True {
                  n253 = call "Get_ADAM_Ch_names_client.vi"("Channel names set"=Channel_names."Active + Off") -> ("Ch names"=w699:string[])
                }
              }
            }
            n254 = call "Get_array_values_fr_String.vi"("String Value"=w669) -> ("String array"=w655:string[])  [unwired: 1 out]
            n255 = Index Array(array=w655, index=0) -> (element=w664:string)
            n256 = Search 1D Array(1D array=w665, element=w664) -> (index of element=w667:i32)  [unwired: 1 out]
            n257 = Index Array(array=w655, index=1) -> (element=w654:string)
            n258 = Empty String/Path?(string/path=w654) -> (empty?=w652:bool)
            n259 = Greater Or Equal To 0?(x=w667) -> (x >= 0?=w666:bool)
            n260 = Select(t="You have not specified a Value to Set the ADAM channel to.\nExample Specifice Argument:  ADAM_Ch_NAME  ;  10", s=w652, f="") -> (s? t:f=w650:string)
            n261 = case shown="False" w666 {
              tunnel: w665 -> [w686 _]
              tunnel: w664 -> [w684 _]
              tunnel: w663 -> [w682 _]
              tunnel: [w680 FALSE ("Cancel")] -> w662
              tunnel: w658 -> [w674 w687]
              tunnel: [w673 w687] -> w657
              tunnel: w654 -> [w671 _]
              frame False {
                n262 = Build Array(w684) -> (w683:string[])
                n263 = Format Into String(format string="Please Select the ADAM Channel that you want to set in row %d", w682) -> (resulting string=w681:string)  [unwired: 2 in, 1 out]
                n264 = call "Select_Strings.vi"("Available Ch names"=w686, "Message"=w681, "Selector mode"=T7."One", "Desired Ch names (in)"=w683) -> ("Cancel"=w680:bool, "Selected Channel Names"=w678:string[])  [unwired: 3 out]
                n265 = Index Array(array=w678, index=0) -> (element=w676:string)
                n266 = Concatenate Strings(w676, "  ;  " ("string"), w671) -> (w672:string)
                n267 = Bundle By Name(cluster=w674, "Specific Arguments"=w672) -> (w673:T1)
              }
              frame True {
              }
            }
            n268 = Select(t="Close Front Panel", s=w662, f=w660) -> (s? t:f=w661:string)
          }
          frame "Run VI Named:" {
            w712 = "Run_VI_Named_specific.vi"
            n269 = Unbundle By Name(w707) -> ("Specific Arguments"=w715:string)
            n270 = global read "Constants_global.vi" "Run VI Folder"() -> (w713:path)
            n271 = Match Pattern(string=w715, regular expression=";") -> (before substring=w716:string)  [unwired: 4 out]
            n272 = call <vilib>:"Trim Whitespace.vi"("string"=w716) -> ("trimmed string"=w708:string)  [unwired: 1 in]
            n273 = call "Run_VI_Named_specific.vi"("Run VI Named String"=w708, "Multi Run Row"=w707) -> ("Checks"=w702:string[], "Error String"=w701:string, "Check for start NaNs?"=w706:bool)  [unwired: 7 out]
            n274 = Select(t="Check for Start NaNs" ("Label for value"), s=w706, f=w704) -> (s? t:f=w703:string)
            n275 = Build Path(base path=w713, name or relative path=w708) -> (appended path=w719:path)
            n276 = Not Equal?(x=w708, y=w712) -> (x != y?=w711:bool)
            n277 = call "Does_file_exist_(simple).vi"("Pathname"=w719) -> ("exists?"=w710:bool)
            n278 = And(x=w710, y=w711) -> (x .and. y?=w709:bool)
            n279 = case shown="False" w709 {
              tunnel: [w726 ""] -> w714
              tunnel: w713 -> [w722 _]
              tunnel: w712 -> [w720 _]
              frame False {
                w724 = "\r"
                n280 = Build Array(w720) -> (w721:string[])
                n281 = call "List_files_in_order_of_age.vi"("Files to Hide"=w721, "Folder"=w722) -> ("file names"=w723:string[])
                n282 = for {
                  shift-right: [w730] -> w727
                  shift-left: "Cannot find the VI to run. Specific Argument options are:" -> [w731]
                  tunnel: w723 -> [w732] mode=indexing
                  w729 = "  " ("Substring")
                  n283 = Concatenate Strings(w731, w729, w732, w729) -> (w730:string)
                }
                n284 = Concatenate Strings(w727, w724, "Please place one of these strings in the \"Specific Argument\" field.", w724) -> (w726:string)
              }
              frame True {
              }
            }
            n285 = Concatenate Strings(w701, w714) -> (w718:string)
          }
          frame "Wait (minutes)" {
            n286 = Unbundle By Name(w735) -> ("Specific Arguments"=w736:string)
            n287 = call "Wait_Case_Arg.vi"("Specific Argument"=w736) -> ("Error Comments"=w737:string)  [unwired: 1 in, 4 out]
          }
          frame "Send Message" {
          }
          frame "Synchronize With:" {
            n288 = local read "Current Sync Number"() -> (w745:i32)
            n289 = call "Synchronize_Prog_Arg.vi"("Execution Row"=w744) -> ("Error Comments"=w747:string, "Sync No"=w753:i32)  [unwired: 3 out]
            n290 = Equal?(x=w753, y=w745) -> (x = y?=w752:bool)
            n291 = Format Into String(format string="This should be Synchroisation number %d.\n" ("Format String"), w745) -> (resulting string=w750:string)  [unwired: 2 in, 1 out]
            n292 = Select(t="", s=w752, f=w750) -> (s? t:f=w748:string)
            n293 = Concatenate Strings(w748, w747) -> (w746:string)
          }
          frame "Fall Back to this Row" {
          }
          frame "Turn Off Row Repeating" {
          }
          frame "Blank Row" {
            n294 = Unbundle By Name(w766) -> ("Comments"=w772:string)
            n295 = Match Pattern(string=w772, regular expression="(No Match Info)") -> (before substring=w765:string, after substring=w769:string)  [unwired: 3 out]
            n296 = Empty String/Path?(string/path=w769) -> (empty?=w770:bool)
            n297 = Bundle By Name(cluster=w766, "Comments"=w765) -> (w764:T1)
            n298 = Select(t=w769, s=w770, f="The Row Type Selector \"%s\" was not matched. Please select the desired type.\n") -> (s? t:f=w768:string)
          }
        }
        "Checks" <- w450
        n299 = Concatenate Strings(w453, w454) -> (w452:string)
      }
      frame "Sort out start and end positions" {
        n300 = Unbundle By Name(w779) -> ("Start X"=w791:dbl, "Start Y"=w790:dbl, "Start Z"=w789:dbl, "End X"=w788:dbl, "End Y"=w787:dbl, "End Z"=w786:dbl, "Extra Commands"=w775:string)
        n301 = call "Which_Trav_Setup.vi"("Extra Command String"=w775) -> ("Traverse Setup"=w774:string)
        n302 = call "Rig_Pict_Display_Pref.vi"("Traverse Name"=w774) -> ("Which Axis is vertical?"=w785:enum16{"X Axis", "Y Axis", "Z Axis"})  [unwired: 7 out]
        n303 = case shown="\"Auto Calibrate\"" w780 {
          tunnel: [w831 FALSE w847 w860 FALSE] -> w794
          tunnel: [w830 FALSE w846 w859 FALSE] -> w793
          tunnel: [w829 FALSE w845 w858 FALSE] -> w792
          tunnel: w785 -> [w828 _ w844 w857 _]
          frame "Vertical Profile" {
            n304 = case shown="\"X Axis\"" w828 {
              tunnel: [FALSE TRUE TRUE] -> w831
              tunnel: [TRUE FALSE TRUE] -> w830
              tunnel: [TRUE TRUE FALSE] -> w829
              frame "X Axis" {
              }
              frame "Y Axis" {
              }
              frame "Z Axis" {
              }
            }
          }
          frame "Auto Calibrate" {
          }
          frame "Lateral Profile" {
            n305 = case shown="\"Y Axis\"" w844 {
              tunnel: [TRUE TRUE TRUE] -> w847
              tunnel: [TRUE TRUE FALSE] -> w846
              tunnel: [FALSE FALSE TRUE] -> w845
              frame "X Axis" {
              }
              frame "Y Axis" {
              }
              frame "Z Axis" {
              }
            }
          }
          frame "Longitudinal Profile" {
            n306 = case shown="\"Y Axis\"" w857 {
              tunnel: [FALSE FALSE FALSE] -> w860
              tunnel: [TRUE TRUE TRUE] -> w859
              tunnel: [TRUE TRUE TRUE] -> w858
              frame "X Axis" {
              }
              frame "Y Axis" {
              }
              frame "Z Axis" {
              }
            }
          }
          frame "Multi-Axis Profile", Default {
          }
        }
        n307 = Build Array(w791, w790, w789) -> (w782:dbl[])
        n308 = Build Array(w788, w787, w786) -> (w781:dbl[])
        n309 = Build Array(w794, w793, w792) -> (w783:bool[])
        "Fixed Axis" <- w783
        n310 = for {
          tunnel: w783 -> [w801] mode=indexing
          tunnel: w782 -> [w800] mode=indexing
          tunnel: w781 -> [w799] mode=indexing
          shift-right: [w796] -> w778
          shift-left: w779 -> [w797]
          i -> [w798]
          n311 = case shown="True" w801 {
            tunnel: w800 -> [_ w807]
            tunnel: w799 -> [_ w806]
            tunnel: w798 -> [_ w805]
            tunnel: w797 -> [w802 w804]
            tunnel: [w802 w803] -> w796
            frame False {
            }
            frame True {
              n312 = Not A Number/Path/Refnum?(number/path/refnum=w807) -> (NaN/Path/Refnum?=w808:bool)
              n313 = Not A Number/Path/Refnum?(number/path/refnum=w806) -> (NaN/Path/Refnum?=w810:bool)
              n314 = Exclusive Or(1:w810, 2:w808) -> (0:w809:bool)
              n315 = case shown="True" w809 {
                tunnel: w808 -> [_ w818]
                tunnel: w807 -> [_ w817]
                tunnel: w806 -> [_ w816]
                tunnel: w805 -> [_ w815]
                tunnel: w804 -> [w811 w814]
                tunnel: [w811 w813] -> w803
                frame False {
                }
                frame True {
                  n316 = Select(t=w816, s=w818, f=w817) -> (s? t:f=w812:dbl)
                  n317 = case shown="2" w815 {
                    tunnel: w814 -> [w821 w824 w827]
                    tunnel: [w820 w823 w826] -> w813
                    tunnel: w812 -> [w819 w822 w825]
                    frame 0, Default {
                      n318 = Bundle By Name(cluster=w821, "Start X"=w819, "End X"=w819) -> (w820:T1)
                    }
                    frame 1 {
                      n319 = Bundle By Name(cluster=w824, "Start Y"=w822, "End Y"=w822) -> (w823:T1)
                    }
                    frame 2 {
                      n320 = Bundle By Name(cluster=w827, "Start Z"=w825, "End Z"=w825) -> (w826:T1)
                    }
                  }
                }
              }
            }
          }
        }
      }
      frame "Check for position NaNs" {
        n321 = global read "Extra_Commands_Global.vi" "Skip Traverse Position Demand"() -> (w876:string)
        n322 = Unbundle By Name(w879) -> ("Extra Commands"=w875:string, "Start X"=w888:dbl, "Start Y"=w886:dbl, "Start Z"=w887:dbl, "End X"=w885:dbl, "End Y"=w884:dbl, "End Z"=w883:dbl)
        n323 = call "Extra_Commands.vi"("String to Search"=w875, "Command"=w876) -> ("Command Found"=w873:bool)  [unwired: 1 in, 4 out]
        n324 = case shown="False" w873 {
          tunnel: w888 -> [w903 _]
          tunnel: w887 -> [w902 _]
          tunnel: w886 -> [w901 _]
          tunnel: w885 -> [w900 _]
          tunnel: w884 -> [w899 _]
          tunnel: w883 -> [w898 _]
          tunnel: [w894 w904] -> w882
          tunnel: [w893 TRUE] -> w881
          tunnel: "" -> [w892 w904]
          frame False {
            n325 = Build Array(w903, w901, w902, w900, w899, w898) -> (w897:dbl[])
            n326 = Not A Number/Path/Refnum?(number/path/refnum=w897) -> (NaN/Path/Refnum?=w896:bool[])
            n327 = Or Array Elements(Boolean array=w896) -> (logical OR=w893:bool)
            n328 = Select(t="Some of the Start and End positions are NaN.\n" ("f"), s=w893, f=w892) -> (s? t:f=w894:string)
          }
          frame True {
          }
        }
        n329 = case shown="\"Set Tunnel Speed Only\", Default" w877 {
          tunnel: w881 -> [_ w910]
          tunnel: ["Check source details" ("t") w909] -> w880
          frame "Multi-Axis Profile" {
          }
          frame "Set Tunnel Speed Only", Default {
            n330 = Select(t="Check source details", s=w910, f="Check profile rows") -> (s? t:f=w909:string)
          }
        }
        n331 = Concatenate Strings(w890, w882) -> (w889:string)
      }
      frame "Check for Start NaNs" {
        n332 = Unbundle By Name(w916) -> ("Extra Commands"=w912:string, "Start X"=w921:dbl, "Start Y"=w919:dbl, "Start Z"=w920:dbl)
        n333 = global read "Extra_Commands_Global.vi" "Skip Traverse Position Demand"() -> (w913:string)
        n334 = call "Extra_Commands.vi"("String to Search"=w912, "Command"=w913) -> ("Command Found"=w911:bool)  [unwired: 1 in, 4 out]
        n335 = case shown="False" w911 {
          tunnel: w921 -> [w933 _]
          tunnel: w920 -> [w932 _]
          tunnel: w919 -> [w931 _]
          tunnel: "" -> [w928 w934]
          tunnel: [w926 w934] -> w917
          frame False {
            n336 = Build Array(w933, w931, w932) -> (w930:dbl[])
            n337 = Not A Number/Path/Refnum?(number/path/refnum=w930) -> (NaN/Path/Refnum?=w929:bool[])
            n338 = Or Array Elements(Boolean array=w929) -> (logical OR=w925:bool)
            n339 = Select(t="Some of the Start coordinates are NaN.\n" ("f"), s=w925, f=w928) -> (s? t:f=w926:string)
          }
          frame True {
          }
        }
        n340 = Concatenate Strings(w923, w917) -> (w922:string)
      }
      frame "Check profile rows" {
        n341 = call "Create_Pos_array.vi"("Traverse line"=w938) -> ("Traverse line Out"=w937:T1, "Error Messages"=w936:string)  [unwired: 7 out]
        n342 = Unbundle By Name(w938) -> ("Start X"=w962:dbl, "Start Y"=w961:dbl, "Start Z"=w960:dbl, "End X"=w959:dbl, "End Y"=w958:dbl, "End Z"=w957:dbl, "Specific Arguments"=w951:string, "Spacing"=w944:T2, "No. of pts."=w943:i32)
        n343 = local read "Fixed Axis"() -> (w942:bool[])
        n344 = Build Array(w962, w961, w960) -> (w940:dbl[])
        n345 = Build Array(w959, w958, w957) -> (w941:dbl[])
        n346 = case shown="\"Specified\"" w944 {
          tunnel: w951 -> [_ _ _ _ w997]
          tunnel: ["" w970 "\"N/A\" is not a valid point spacing.\n" "" w992] -> w950
          tunnel: w943 -> [_ _ _ _ w996]
          tunnel: w942 -> [_ w968 _ _ _]
          tunnel: w941 -> [_ w975 _ _ _]
          tunnel: w940 -> [_ w974 _ _ _]
          frame "Linear" {
          }
          frame "Log" {
            n347 = for {
              tunnel: w975 -> [w979] mode=indexing
              tunnel: w974 -> [w978] mode=indexing
              tunnel: [w977] -> w973 mode=indexing
              tunnel: w968 -> [w976] mode=indexing
              n348 = case shown="False" w976 {
                tunnel: w979 -> [w985 _]
                tunnel: w978 -> [w984 _]
                tunnel: [w980 FALSE] -> w977
                frame False {
                  w983 = 0.001 ("y")
                  n349 = Less?(x=w985, y=w983) -> (x < y?=w981:bool)
                  n350 = Less?(x=w984, y=w983) -> (x < y?=w982:bool)
                  n351 = Or(x=w981, y=w982) -> (x .or. y?=w980:bool)
                }
                frame True {
                }
              }
            }
            n352 = Or Array Elements(Boolean array=w973) -> (logical OR=w972:bool)
            n353 = Select(t="For log spacing, Start & End positions must be greater than 0.0001.", s=w972, f="") -> (s? t:f=w970:string)
          }
          frame "N/A" {
          }
          frame "Gauss" {
          }
          frame "Specified" {
            n354 = call "Get_array_values_fr_String.vi"("String Value"=w997) -> ("Numeric Array"=w991:dbl[])  [unwired: 1 out]
            n355 = Array Size(array=w991) -> (size(s)=w990:i32)
            n356 = Decrement(x=w990) -> (x-1=w989:i32)
            n357 = Equal?(x=w989, y=w996) -> (x = y?=w995:bool)
            n358 = Select(t="", s=w995, f="The No of points and No of Arguments do not match.\n") -> (s? t:f=w992:string)
          }
        }
        n359 = for {
          tunnel: w942 -> [w1002] mode=indexing
          tunnel: w940 -> [w1001] mode=indexing
          tunnel: w941 -> [w1000] mode=indexing
          tunnel: [w999] -> w956 mode=indexing
          tunnel: [w998] -> w947 mode=indexing
          n360 = case shown="False" w1002 {
            tunnel: w1001 -> [w1004 w1010]
            tunnel: w1000 -> [w1005 w1009]
            tunnel: [TRUE w1008] -> w999
            tunnel: [w1003 TRUE] -> w998
            frame False {
              n361 = Not Equal?(x=w1004, y=w1005) -> (x != y?=w1003:bool)
            }
            frame True {
              n362 = Equal?(x=w1010, y=w1009) -> (x = y?=w1008:bool)
            }
          }
        }
        n363 = And Array Elements(Boolean array=w956) -> (logical AND=w955:bool)
        n364 = Or Array Elements(Boolean array=w947) -> (logical OR=w948:bool)
        n365 = Select(t="", s=w955, f="This profile moves more than one axis.\n") -> (s? t:f=w952:string)
        n366 = Select(t="", s=w948, f="The start and end points are the same for this profile.\n") -> (s? t:f=w946:string)
        n367 = Concatenate Strings(w936, w946, w952, w950) -> (w965:string)
        n368 = Concatenate Strings(w964, w965) -> (w963:string)
      }
      frame "Check source details" {
        n369 = Unbundle By Name(w1022) -> ("Emission Rate (l/min)"=w1024:dbl, "Density Ratio"=w1014:string)  [unwired: 1 out]
        n370 = Empty String/Path?(string/path=w1014) -> (empty?=w1015:bool)
        n371 = Equal?(x=w1014, y="---------" ("f")) -> (x = y?=w1013:bool)
        n372 = Or(x=w1015, y=w1013) -> (x .or. y?=w1012:bool)
        n373 = Greater Than 0?(x=w1024) -> (x > 0?=w1019:bool)
        n374 = And(x=w1019, y=w1012) -> (x .and. y?=w1023:bool)
        n375 = case shown="True" w1023 {
          tunnel: w1022 -> [w1027 w1030]
          tunnel: [w1027 w1028] -> w1021
          frame False {
          }
          frame True {
            (unwired) "The Density Ratio Box should contain either:\nCarrier 1 Only\nCarrier 2 Only\nor the relative density ratio of the mixed gas with respect to air" ("f")
            n376 = Bundle By Name(cluster=w1030, "Density Ratio"="Carrier 1 Only") -> (w1028:T1)
          }
        }
        n377 = Select(t="Check source detail 2", s=w1019, f="check entered filename etc") -> (s? t:f=w1017:string)
      }
      frame "Check source detail 2" {
        n378 = Unbundle By Name(w1054) -> ("Trace Gas Concentration (%)"=w1055:dbl, "Density Ratio"=w1056:string)
        n379 = To Upper Case(1:w1056) -> (0:w1039:string)
        n380 = To Upper Case(1:"Carrier 1 Only") -> (0:w1041:string)
        n381 = To Upper Case(1:"Carrier 2 Only") -> (0:w1040:string)
        n382 = In Range and Coerce(upper limit=ext 3.01 ("hi"), x=w1055, lower limit=ext 0.0 ("lo")) -> (In Range?=w1036:bool)  [unwired: 1 out]
        n383 = Equal?(x=w1039, y=w1041) -> (x = y?=w1046:bool)
        n384 = Equal?(x=w1039, y=w1040) -> (x = y?=w1045:bool)
        n385 = Fract/Exp String To Number(string=w1039) -> (number=w1047:dbl)  [unwired: 4 out]
        n386 = In Range and Coerce(upper limit=ext 10.0 ("hi"), x=w1047, lower limit=ext 0.05 ("lo")) -> (In Range?=w1044:bool)  [unwired: 1 out]
        n387 = Compound Arithmetic op=OR(w1046, w1045, w1044) -> (w1031:bool)
        n388 = Select(t="", s=w1036, f="The Trace Gas Concentration must be within the range of 0 to 3%.\n") -> (s? t:f=w1032:string)
        n389 = Select(t="", s=w1031, f="The Density Ratio Box should contain either:\nCarrier 1 Only\nCarrier 2 Only\nor the relative density ratio of the mixed gas with respect to air") -> (s? t:f=w1033:string)
        n390 = Concatenate Strings(w1032, w1033) -> (w1057:string)
        n391 = Concatenate Strings(w1059, w1057) -> (w1058:string)
      }
      frame "check entered filename etc" {
        n392 = local read "Checks"() -> (w1072:string[])
        n393 = for {
          tunnel: w1072 -> [w1079] mode=indexing
          tunnel: [w1084] -> w1073 mode=indexing
          tunnel: w1069 -> [w1083]
          shift-right: [w1081] -> w1063
          shift-left: w1064 -> [w1082]
          tunnel: [w1080] -> w1062 mode=indexing
          n394 = case shown="\"Filename:HD:Users\"" w1079 {
            tunnel: w1082 -> [w1086 w1094 w1116 w1131]
            tunnel: [w1087 w1097 w1122 w1127] -> w1084
            tunnel: w1083 -> [_ _ w1125 _]
            tunnel: [w1086 w1094 w1114 w1131] -> w1081
            tunnel: [TRUE ("cancelled") TRUE ("cancelled") w1109 TRUE ("cancelled")] -> w1080
            tunnel: w1079 -> [_ _ _ w1129]
            frame "Number:Of:Points" {
              n395 = Unbundle By Name(w1086) -> ("No. of pts."=w1089:i32)
              n396 = Greater?(x=w1089, y=1) -> (0:w1091:bool)
              n397 = Select(t="", s=w1091, f="For a profile the number of points should be more than 1.\n" ("Format String")) -> (s? t:f=w1087:string)
            }
            frame "Averaging:Time:(mins)" {
              n398 = Unbundle By Name(w1094) -> ("Averaging time (min)"=w1096:dbl)
              n399 = Greater Than 0?(x=w1096) -> (x > 0?=w1095:bool)
              n400 = Select(t="", s=w1095, f="The averaging time should be greater than zero.\n" ("Format String")) -> (s? t:f=w1097:string)
            }
            frame "Filename:HD:Users" {
              w1123 = FALSE  # Show Error handler
              n401 = Unbundle By Name(w1116) -> ("Filename"=w1100:path, "Row No"=w1111:i32, "Row Type Selector"=w1107:T3)
              n402 = call "Row_type_selector_string.vi"("Mode"=w1107) -> ("Output string"=w1106:string)
              n403 = call "Current_Filepath.vi"("Filename in"=w1100, "Data Type"="Results") -> ("Filename Out"=w1101:path)  [unwired: 1 out]
              n404 = Path To String(path=w1101) -> (string=w1120:string)
              n405 = Not A Number/Path/Refnum?(number/path/refnum=w1101) -> (NaN/Path/Refnum?=w1104:bool)
              n406 = Equal?(x=Multi_run_mode."Run VI Named:" ("Mode"), y=w1125) -> (x = y?=w1124:bool)
              n407 = Match Pattern(string=w1120, regular expression="-------" ("f")) -> (match substring=w1119:string)  [unwired: 4 out]
              n408 = Empty String/Path?(string/path=w1119) -> (empty?=w1105:bool)
              n409 = Format Into String(format string=" For Row  %d %s." ("Comment"), w1111, w1106) -> (resulting string=w1110:string)  [unwired: 2 in, 1 out]
              n410 = Compound Arithmetic op=AND(w1105, invert w1104) -> (w1103:bool)
              n411 = Select(t=w1101, s=w1103, f=path "") -> (s? t:f=w1118:path)
              n412 = call "Results_filename_checker.vi"("Filelength"=35, "Warn if Already Exists"=w1124, "Comment"=w1110, "Show Error handler"=w1123, "Results file"=w1118) -> ("Error String"=w1122:string, "cancelled"=w1113:bool, "Results file output"=w1115:path)  [unwired: 1 out]
              n413 = Bundle By Name(cluster=w1116, "Filename"=w1115) -> (w1114:T1)
              n414 = Not(x=w1113) -> (.not. x?=w1109:bool)
            }
            frame "No Match", Default {
              n415 = Concatenate Strings(w1129, " Has not been programmed.\n" ("string")) -> (w1127:string)
            }
          }
        }
        n416 = local read "Editted Row"() -> (w1066:bool)
        n417 = And Array Elements(Boolean array=w1062) -> (logical AND=w1061:bool)
        n418 = Concatenate Strings(w1073) -> (w1071:string)
        n419 = Concatenate Strings(w1070, w1071) -> (w1065:string)
        n420 = Empty String/Path?(string/path=w1065) -> (empty?=w1068:bool)
        n421 = case shown="True" w1068 {
          tunnel: ["Open Front Panel" w1077] -> w1067
          tunnel: w1066 -> [_ w1078]
          frame False {
          }
          frame True {
            n422 = Select(t="Close Front Panel", s=w1078, f="End") -> (s? t:f=w1077:string)
          }
        }
      }
      frame "Open Front Panel" {
        w1136 = TRUE  # Front Panel Window:Open
        n423 = Current VI's Path() -> (path=w1137:path)
        n424 = call "Open_Close_Front_Panel.ph.vi"("Front Panel Window:Open"=w1136, "VI path"=w1137) -> ()  [unwired: 2 out]
        n425 = local write "Editted Row"(TRUE ("Editted Row")) -> ()
        n426 = local write "Execution Row"(w1133) -> ()
      }
      frame "What to do next?" {
        w1147 = ""
        w1145 = "[\r\n]"
        n427 = local read "Execution Row"() -> (w1143:T1)
        n428 = Unbundle By Name(w1143) -> ("Row Type Selector"=w1159:T3, "Specific Arguments"=w1154:string, "Extra Commands"=w1152:string, "Density Ratio"=w1146:string)
        n429 = Wait Until Next ms Multiple(millisecond multiple=u32 100) -> ()  [unwired: 1 out]
        n430 = Not Equal?(x=Multi_run_mode."Blank Row" ("Mode"), y=w1159) -> (x != y?=w1155:bool)
        n431 = call "Replace_Character.vi"("Replace with"=w1147, "Input String"=w1154, "Search For"=w1145) -> ("Output string"=w1153:string)  [unwired: 1 out]
        n432 = call "Replace_Character.vi"("Replace with"=w1147, "Input String"=w1152, "Search For"=w1145) -> ("Output string"=w1151:string)  [unwired: 1 out]
        n433 = call "Replace_Character.vi"("Replace with"=w1147, "Input String"=w1146, "Search For"=w1145) -> ("Output string"=w1144:string)  [unwired: 1 out]
        n434 = Compound Arithmetic op=OR("Edit in Excel", "OK") -> (w1156:bool)
        n435 = Bundle By Name(cluster=w1143, "Specific Arguments"=w1153, "Extra Commands"=w1151, "Density Ratio"=w1144) -> (w1141:T1)
        n436 = Compound Arithmetic op=AND(w1156, w1155) -> (w1149:bool)
        n437 = Not Equal?(x=w1141, y=w1143) -> (x != y?=w1142:bool)
        n438 = Not(x="Edit in Excel") -> (.not. x?=w1140:bool)
        n439 = case shown="True" w1142 {
          tunnel: w1141 -> [_ w1163]
          frame False {
          }
          frame True {
            n440 = local write "Execution Row"(w1163) -> ()
          }
        }
        n441 = case shown="False" w1140 {
          tunnel: ["Close Front Panel" w1168] -> w1148
          tunnel: w1149 -> [_ w1167]
          frame False {
          }
          frame True {
            n442 = Select(t="Clean Up Row", s=w1167, f="What to do next?") -> (s? t:f=w1168:string)
          }
        }
        "Error Comments" <- w1150
      }
      frame "Clean Up Row" {
        n443 = call "Traverse_Control_Ch_Names.vi"("Mode"=T4."All Channel Names") -> ("Channel names"=w1177:string[])  [unwired: 1 in]
        n444 = call "Trav_Cluster_to_Row.vi"("Traverse line in"=w1172, "Row Number"=w1173, "Channel names"=w1177) -> ("Traverse line Out"=w1175:T1)  [unwired: 4 out]
      }
      frame "Close Front Panel" {
        w1181 = FALSE  # Front Panel Window:Open
        n445 = Current VI's Path() -> (path=w1182:path)
        n446 = call "Open_Close_Front_Panel.ph.vi"("Front Panel Window:Open"=w1181, "VI path"=w1182) -> ()  [unwired: 2 out]
      }
      frame "End" {
        n447 = local read "Editted Row"() -> (w1190:bool)
        n448 = case shown="True" w1190 {
          tunnel: w1189 -> [w1193 w1196]
          tunnel: [w1193 w1195] -> w1187
          tunnel: w1188 -> [_ w1194]
          frame False {
          }
          frame True {
            n449 = call "Traverse_Control_Ch_Names.vi"("Mode"=T4."All Channel Names") -> ("Channel names"=w1197:string[])  [unwired: 1 in]
            n450 = call "Trav_Cluster_to_Row.vi"("Traverse line in"=w1196, "Row Number"=w1194, "Channel names"=w1197) -> ("Traverse line Out"=w1195:T1)  [unwired: 4 out]
          }
        }
        n451 = local write "Error Comments"(w1191) -> ()
      }
    }
  }
  "Execution Row Out" <- w2
  "Continue?" <- w1
